vi "PXI_Host_U32_Write_NewMethod_Benchmark.vi"() -> ()   [LabVIEW 2018]
uses:
  <vilib>/Platform/TimedLoop/XDataNode/timing_clust.ctl
  <vilib>/Platform/TimedLoop/XDataNode/nitl_modes.ctl
  <vilib>/Platform/TimedLoop/XDataNode/wakeup.ctl
  cRIO RT/FPGA Bitfile Register Operations/Scalar IO Operations/Write Methods/Write Data Register/Instances/Write U32.vi
  cRIO RT/FPGA Bitfile Register Operations/Scalar IO Operations/Utilities/Find Register Offset.vi
  cRIO RT/FPGA Bitfile Register Operations/Scalar IO Operations/SubVIs/Check Register Data Store.vi
  cRIO RT/FPGA Bitfile Register Operations/Scalar IO Operations/Error Handling/Error 6001.vi
  cRIO RT/FPGA Bitfile Register Operations/Scalar IO Operations/Error Handling/Error 6000.vi
  cRIO RT/FPGA Bitfile Register Operations/Scalar IO Operations/Error Handling/Error 6002.vi
  cRIO RT/FPGA Bitfile Register Operations/Scalar IO Operations/Error Handling/Error 6006.vi
  <vilib>/FPGAPlugInAG/Dynamic/niLvFpga_Close_Dynamic.vi
  <vilib>/platform/TimedLoop/XDataNode/XDataNode.xnode
  <vilib>/rvi/interface/nirviCloseFPGA/nirviCloseFPGA.xnode
  cRIO RT/FPGA Bitfile Register Operations/Scalar IO Operations/FPGA Register IO.lvlib
  <vilib>/Platform/TimedLoop/XDataNode/XDNodeRunTimeDep.lvlib
panel:
  out "Maximum(s)":dbl
  out "Standard deviation":dbl
  out "Waveform Graph":dbl[](graph)
  out "error out":errorcluster
  out "Execution time (s)":dbl
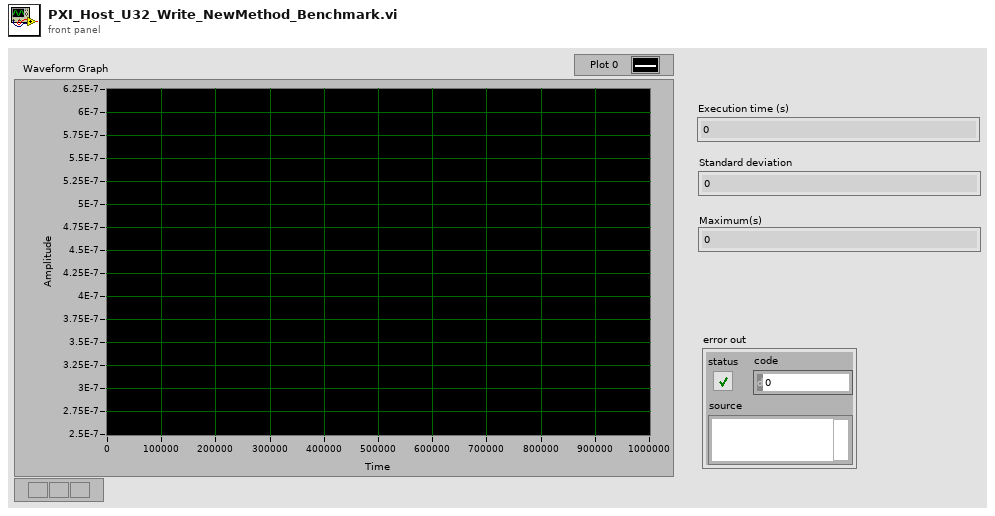
[diagram p1: front panel]
types:
  T1 = typedef "XDNodeRunTimeDep.lvlib/timing_clust.ctl" = cluster{"Expected End [f-1]":u64, "Actual End [f-1]":u64, "Finished Late? [f-1]":bool, "Expected End [i-1]":u64, "Actual End [i-1]":u64, "Finished Late? [i-1]":bool, "Expected Start [i]":u64, "Actual Start [i]":u64, "Expected Start [f]":u64, "Actual Start [f]":u64, "Source Name":string, "Structure Name":string, "Period":i64, "Deadline":i64, "Offset":i64, "Start":i64, "Priority":i32, "Timeout":i32, "Mode":T2, "Wakeup Reason":T3, "Error":errorcluster, "Source Type":string, "Secondary Source Type":string, "Global End Time":u64, "Global Start Time":u64, "Frame Duration":u64, "Iteration Duration":u64, "Assigned CPU":i32, "I/O Scan Engine Mode":u32}
  T2 = typedef "XDNodeRunTimeDep.lvlib/nitl_modes.ctl" = enum32{"No Change", "Process missed periods, maintain original phase", "Discard missed periods, maintain original phase", "Process missed periods, ignore original phase", "Discard missed periods, ignore original phase"}
  T3 = typedef "XDNodeRunTimeDep.lvlib/wakeup.ctl" = enum32{"Normal", "Aborted", "Asynchronous wakeup", "Timing source error", "Timed loop error", "Timeout"}
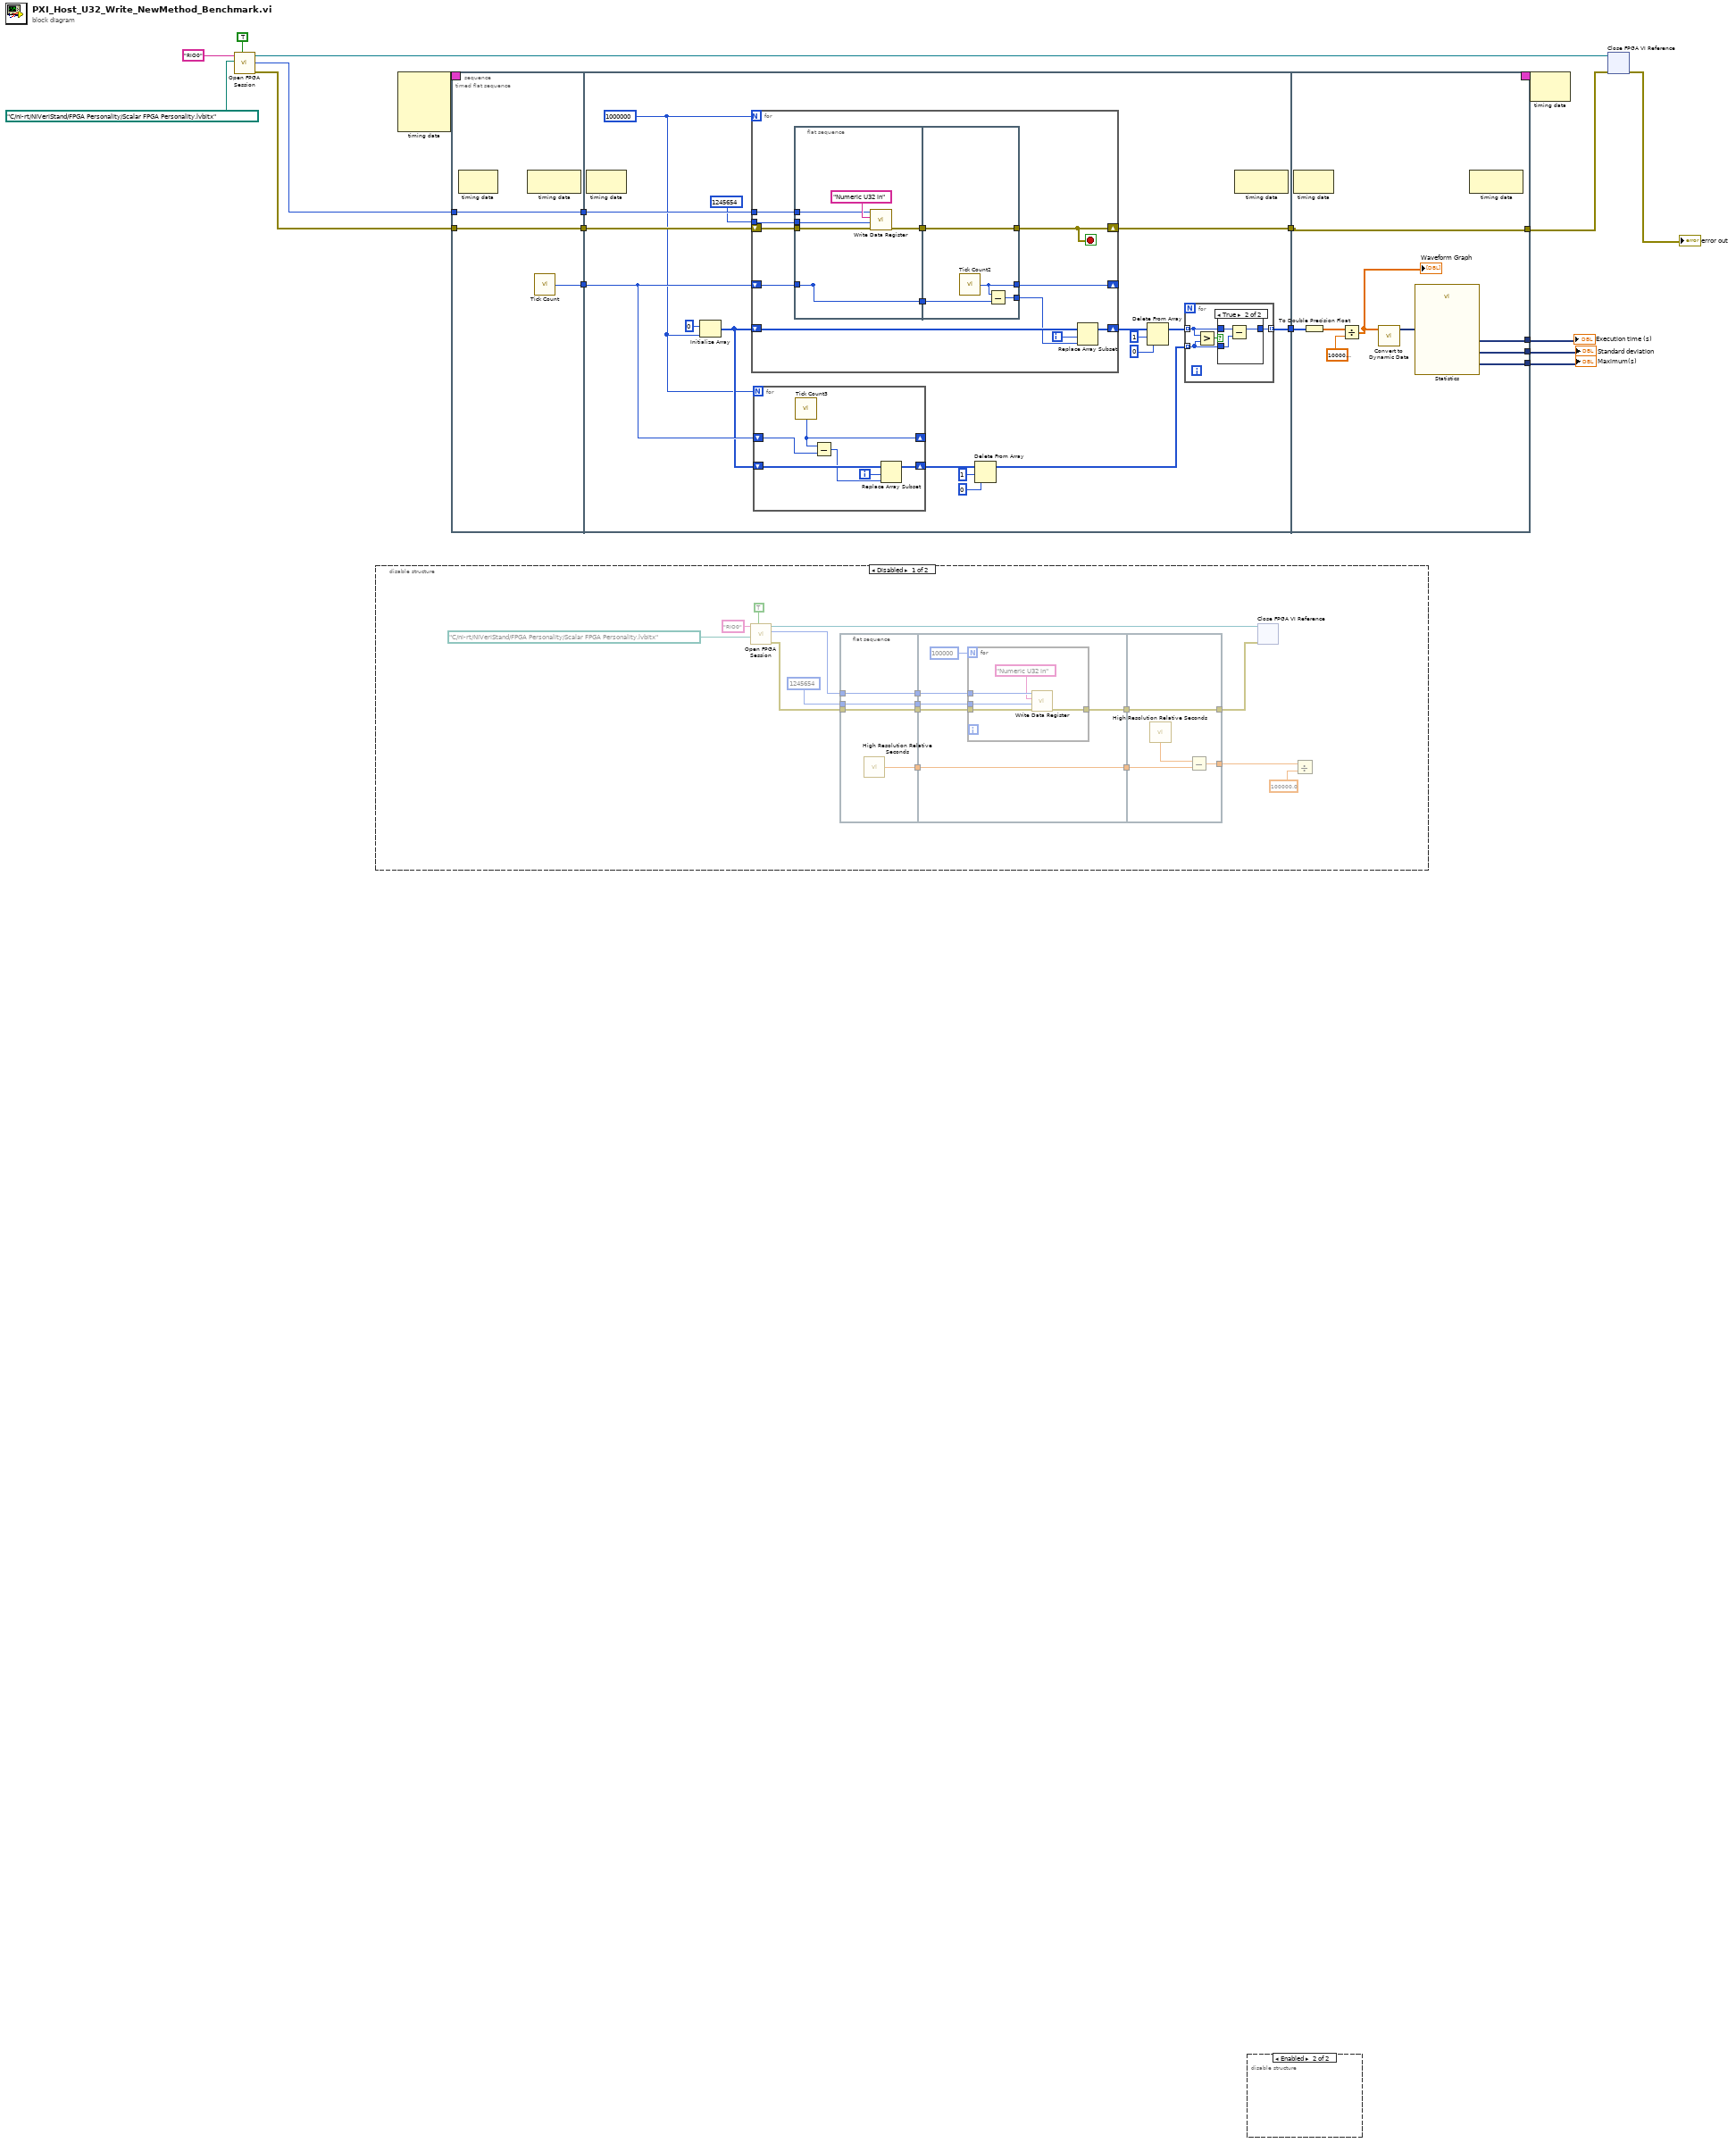
[diagram p0: block diagram]
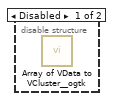
[diagram p4: hidden frame]
diagram:
  n1 = call "Open FPGA Session.vi"("run when loaded (T)"=TRUE, "bitfile path"=path "C:/ni-rt/NIVeriStand/FPGA Personality/Scalar FPGA Personality.lvbitx", "device address"="RIO0") -> ("error out"=w7:errorcluster, "session out"=w11:u32, "bitfile reference out"=w6:refnum<k20>)  [unwired: 6 in]
  n2 = disable-structure shown="Disabled" {
    frame Disabled {
      n3 = call "Open FPGA Session.vi"("run when loaded (T)"=TRUE, "bitfile path"=path "C:/ni-rt/NIVeriStand/FPGA Personality/Scalar FPGA Personality.lvbitx", "device address"="RIO0") -> ("error out"=w17:errorcluster, "session out"=w21:u32, "bitfile reference out"=w16:refnum<k20>)  [unwired: 6 in]
      n4 = flat-sequence {
        tunnel: [w33] -> w29
        tunnel: w21 -> [w32]
        tunnel: [w32] -> w28
        tunnel: w17 -> [w31]
        tunnel: [w31] -> w27
        tunnel: [w30] -> w26
        tunnel: u32 1245654 ("value in") -> [w30]
        tunnel: [w38] -> w25
        tunnel: w29 -> [w38]
        tunnel: w28 -> [w37]
        tunnel: w27 -> [w36]
        tunnel: [w35] -> w24
        tunnel: w26 -> [w34]
        tunnel: w25 -> [w47]
        tunnel: [w46] -> w23
        tunnel: w24 -> [w45]
        tunnel: [w45] -> w15
        frame #0 {
          n5 = call <vilib>:"High Resolution Relative Seconds.vi"() -> ("relative seconds"=w33:dbl)
        }
        frame #1 {
          n6 = for {
            N: 100000 -> [_]
            tunnel: w37 -> [w42]
            tunnel: w36 -> [w43]
            tunnel: [w44] -> w35
            tunnel: w34 -> [w40]
            n7 = call-poly "Write Data Register.vi"("error in"=w43, "value in"=w40, "register name"="Numeric U32 in", "session in"=w42) -> ("error out"=w44:errorcluster)  [unwired: 6 in, 1 out]
          }
        }
        frame #2 {
          n8 = call <vilib>:"High Resolution Relative Seconds.vi"() -> ("relative seconds"=w48:dbl)
          n9 = Subtract(x=w48, y=w47) -> (x-y=w46:dbl)
        }
      }
      n10 = xnode "Close FPGA VI Reference"("FPGA VI Reference In"=w16, "error in"=w15) -> ()  [unwired: 1 out]
      n11 = Divide(x=w23, y=100000.0) -> ()  [unwired: 1 out]
    }
    frame Enabled {
    }
  }
  n12 = node-c288() -> (w13:T1)  [unwired: 4 in]
  n13 = timed-sequence {
    timing: w13 -> [_]
    timing-out: [_] -> w12
    tunnel: w11 -> [w59]
    tunnel: w7 -> [w58]
    tunnel: [w54] -> w5
    tunnel: [w52] -> w3
    tunnel: [w51] -> w2
    tunnel: [w50] -> w1
    n14 = timed-flat-sequence {
      tunnel: w59 -> [w62]
      tunnel: [w62] -> w57
      tunnel: w58 -> [w61]
      tunnel: [w61] -> w56
      tunnel: [w60] -> w53
      tunnel: w57 -> [w81]
      tunnel: w56 -> [w80]
      tunnel: [w79] -> w55
      tunnel: w53 -> [w73]
      tunnel: [w66] -> w49
      tunnel: w55 -> [w128]
      tunnel: [w128] -> w54
      tunnel: [w126] -> w52
      tunnel: [w123] -> w51
      tunnel: [w122] -> w50
      tunnel: w49 -> [w121]
      frame #0 {
        n15 = node-c288() -> ()  [unwired: 1 in, 1 out]
        n16 = node-c288() -> ()  [unwired: 1 in, 1 out]
        n17 = call "Tick Count"() -> ("Tick Count(Ticks)"=w60:u32)
      }
      frame #1 {
        w68 = 1000000
        n18 = node-c288() -> ()  [unwired: 1 in, 1 out]
        n19 = Initialize Array(u32 0, w68) -> (w72:u32[])
        n20 = for {
          N: w68 -> [_]
          tunnel: w81 -> [w108]
          shift-right: [w106] -> _
          shift-left: w73 -> [w105]
          shift-right: [w101] -> w77
          shift-left: w72 -> [w103]
          shift-right: [w99] -> w79
          shift-left: w80 -> [w109]
          tunnel: u32 1245654 ("value in") -> [w98]
          i -> [w100]
          stop <- w99 stop-if-true
          n21 = flat-sequence {
            tunnel: w109 -> [w113]
            tunnel: w108 -> [w111]
            tunnel: [w112] -> w107
            tunnel: [w115] -> _
            tunnel: w105 -> [w115]
            tunnel: [w115] -> w104
            tunnel: w98 -> [w110]
            tunnel: [w119] -> w99
            tunnel: w107 -> [w119]
            tunnel: [w118] -> w106
            tunnel: w104 -> [w117]
            tunnel: [w116] -> w102
            frame #0 {
              n22 = call-poly "Write Data Register.vi"("error in"=w113, "value in"=w110, "register name"="Numeric U32 in", "session in"=w111) -> ("error out"=w112:errorcluster)  [unwired: 6 in, 1 out]
            }
            frame #1 {
              n23 = call "Tick Count2"() -> ("Tick Count(Ticks)"=w118:u32)
              n24 = Subtract(x=w118, y=w117) -> (x-y=w116:u32)
            }
          }
          n25 = Replace Array Subset(array=w103, new element=w102, index=w100) -> (w101:u32[])
        }
        n26 = for {
          N: w68 -> [_]
          shift-right: [w90] -> w69
          shift-left: w72 -> [w93]
          shift-right: [w95] -> _
          shift-left: w73 -> [w94]
          i -> [w91]
          n27 = call "Tick Count3"() -> ("Tick Count(Ticks)"=w95:u32)
          n28 = Subtract(x=w95, y=w94) -> (x-y=w92:u32)
          n29 = Replace Array Subset(array=w93, new element=w92, index=w91) -> (w90:u32[])
        }
        n30 = Delete From Array(array=w69, length=1, index=0) -> (array with subset deleted=w65:u32[])  [unwired: 1 out]
        n31 = Delete From Array(array=w77, length=1, index=0) -> (array with subset deleted=w67:u32[])  [unwired: 1 out]
        n32 = for {
          tunnel: [w85] -> w66 mode=indexing
          tunnel: w67 -> [w84] mode=indexing
          tunnel: w65 -> [w83] mode=indexing
          n33 = Greater?(x=w84, y=w83) -> (0:w82:bool)
          n34 = case shown="True" w82 {
            tunnel: w84 -> [w86 w89]
            tunnel: w83 -> [_ w88]
            tunnel: [w86 w87] -> w85
            frame False {
            }
            frame True {
              n35 = Subtract(x=w89, y=w88) -> (x-y=w87:u32)
            }
          }
        }
        n36 = node-c288() -> ()  [unwired: 1 in, 1 out]
      }
      frame #2 {
        n37 = node-c288() -> ()  [unwired: 1 in, 1 out]
        n38 = To Double Precision Float(number=w121) -> (double precision float=w125:dbl[])
        n39 = Divide(x=w125, y=1000000000.0) -> (x/y=w120:dbl[])
        "Waveform Graph" <- w120
        n40 = call "Convert to Dynamic Data"("Array"=w120) -> ("Dynamic Data Type"=w127:dynamicdata)  [unwired: 3 in]
        n41 = call "Statistics"("Signals"=w127) -> ("Standard Dev"=w123:dynamicdata, "Arithmetic Mean"=w126:dynamicdata, "Maximum"=w122:dynamicdata)  [unwired: 23 in, 1 out]
        n42 = node-c288() -> ()  [unwired: 1 in, 1 out]
      }
    }
  }
  "Execution time (s)" <- w3
  "Standard deviation" <- w2
  "Maximum(s)" <- w1
  n43 = disable-structure shown="Enabled" {
    frame Disabled {
      n44 = call <userlib>:"Array of VData to VCluster__ogtk.vi"() -> ()  [unwired: 10 in, 2 out]
    }
    frame Enabled {
    }
  }
  n45 = node-c288(w12) -> ()  [unwired: 1 out]
  n46 = xnode "Close FPGA VI Reference"("FPGA VI Reference In"=w6, "error in"=w5) -> ("error out"=→"error out":errorcluster)
